vi "TestPostDCIR.vi"(7 "Variante":string, 8 "errin":errorcluster, 10 "3P4S?":bool, 11 "isPASS?":bool) -> (0 "errout":errorcluster, 1 "message box":string, 2 "taboutBdd":string[](array[string]), 3 "test OK?":bool, 4 "Chaîne 2":string, 5 "offprbarre":bool)   [LabVIEW 2020]
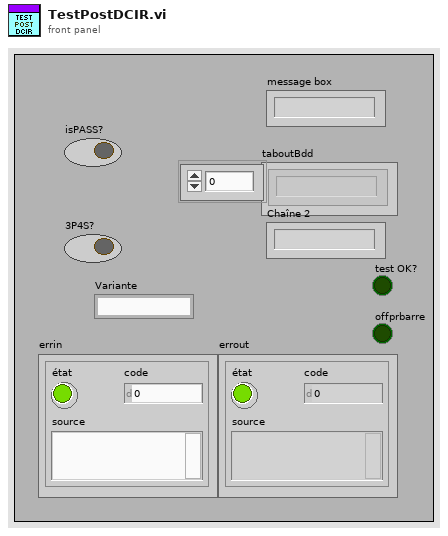
[diagram p1: front panel]
types:
  T1 = cluster{"Cell1 V":sgl, "Cell2 V":sgl, "Cell3 V":sgl, "Cell4 V":sgl, "Cell1 °C":sgl, "Cell2 °C":sgl, "Cell5 V":sgl, "Cell6 V":sgl}
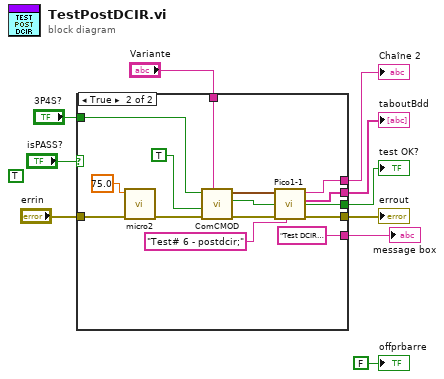
[diagram p0: block diagram]
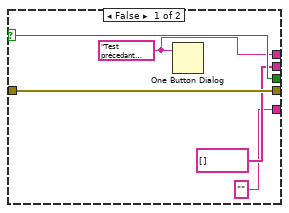
[diagram p2: hidden frame]
diagram:
  (unwired) TRUE
  n1 = case shown="True" "isPASS?" {
    selector: "isPASS?" -> [w15 _]
    tunnel: [w15 w28] -> w4
    tunnel: [w13 w26] -> w6
    tunnel: "errin" -> [w14 w24]
    tunnel: [w14 w25] -> w5
    tunnel: [string[] [] ("tableau ajouté") w20] -> w8
    tunnel: "3P4S?" -> [_ w19]
    tunnel: ["" ("Chaîne") "Test DCIR: Lecture des Cell2" ("Chaîne")] -> w10
    tunnel: "Variante" -> [_ w16]
    frame False {
      w13 = "Test précedant (DCIR) FAIL" ("Chaîne")
      n2 = One Button Dialog(message=w13) -> ()  [unwired: 1 in, 1 out]
    }
    frame True {
      n3 = call "micro2.vi"("errin"=w24, "offset%"=75.0) -> ("errout"=w23:errorcluster)  [unwired: 9 in]
      n4 = call "ComCMOD.vi"("Variante"=w16, "errin"=w23, "PostDCIR ?"=TRUE, "3P4S"=w19) -> ("errout"=w25:errorcluster, "test OK?"=w28:bool, "Out"=w27:T1)  [unwired: 5 in]
      n5 = call "Pico1-1.vi"("ajout test#"="Test# 6 - postdcir;", "Datain"=w27) -> ("taboutBdd"=w20:string[], "Chaîne"=w26:string)  [unwired: 8 in]
    }
  }
  "message box" <- w10
  "taboutBdd" <- w8
  "Chaîne 2" <- w6
  "errout" <- w5
  "test OK?" <- w4
  "offprbarre" <- FALSE
